vi "Generate Command Sequence.vi"() -> ()   [LabVIEW 2019]
uses:
  Controls/Command Sequene Control.ctl
panel:
  out "error out":errorcluster
  out "File path":path
  in  "Path Name":string
  out "Command Sequence":string
  in  "Auto Control":T1
  in  "Generate Path":bool
  in  "Add Command":bool
  in  "stop":bool
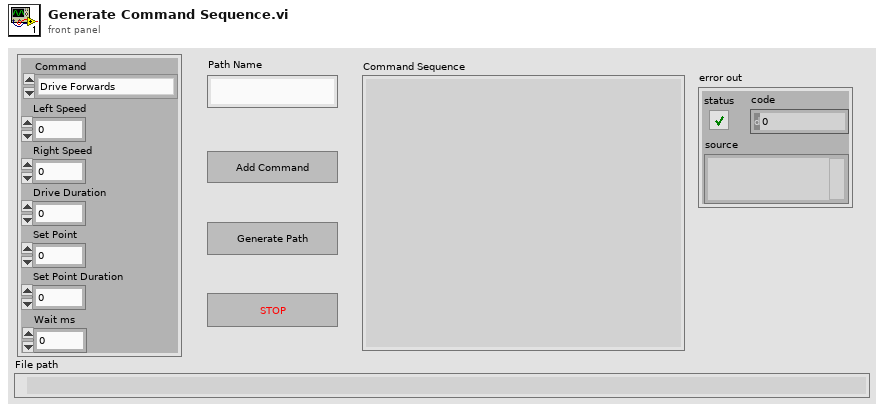
[diagram p1: front panel]
types:
  T1 = cluster{"Drive Duration":dbl, "Left Speed":dbl, "Right Speed":dbl, "Set Point":dbl, "Set Point Duration":dbl, "Command":enum16{"Drive Forwards", "Drive Backwards", "Stop", "Turn Left", "Turn Right", "Drop Intake", "Lift Intake", "Intake", "Shooter", "Transfer", "Wait"}, "Wait ms":dbl}
  T2 = typedef "Command Sequene Control.ctl" = enum16{"Idle", "Stop", "Add command", "Create Path File", "Check File Name"}
  T3 = enum16{"open", "replace", "create", "open or create", "replace or create", "replace or create with confirmation"}
  T4 = enum16{"Drive Forwards", "Drive Backwards", "Stop", "Turn Left", "Turn Right", "Drop Intake", "Lift Intake", "Intake", "Shooter", "Transfer", "Wait"}
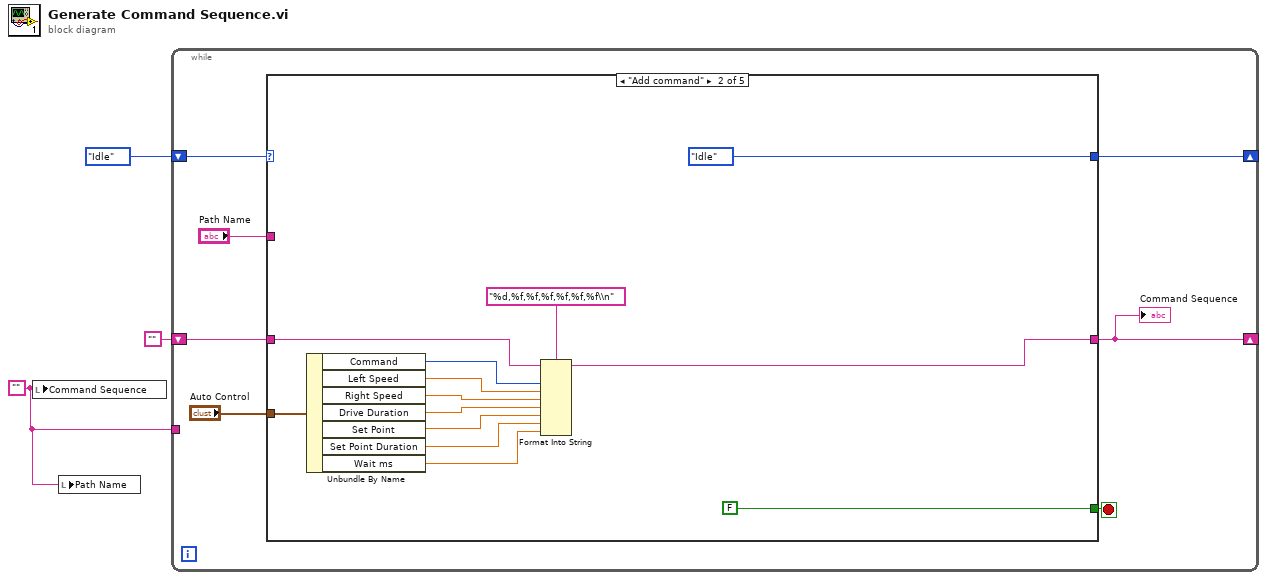
[diagram p0: block diagram]
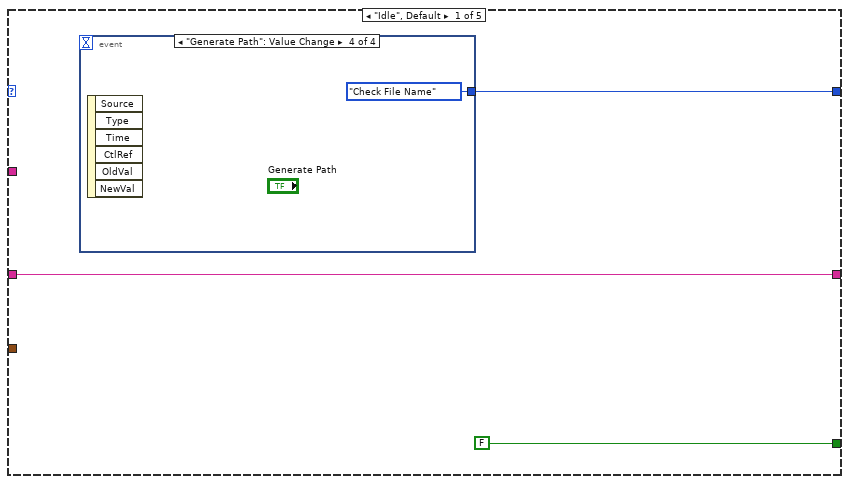
[diagram p2: hidden frame]
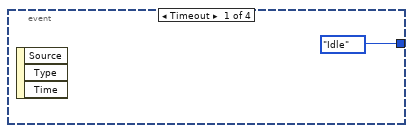
[diagram p3: hidden frame]
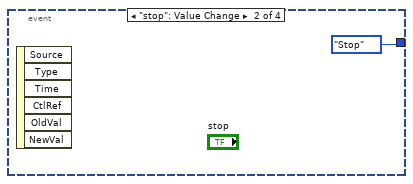
[diagram p4: hidden frame]
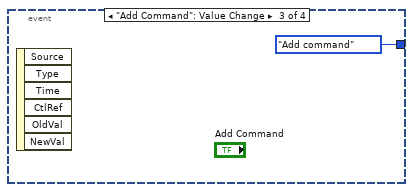
[diagram p5: hidden frame]
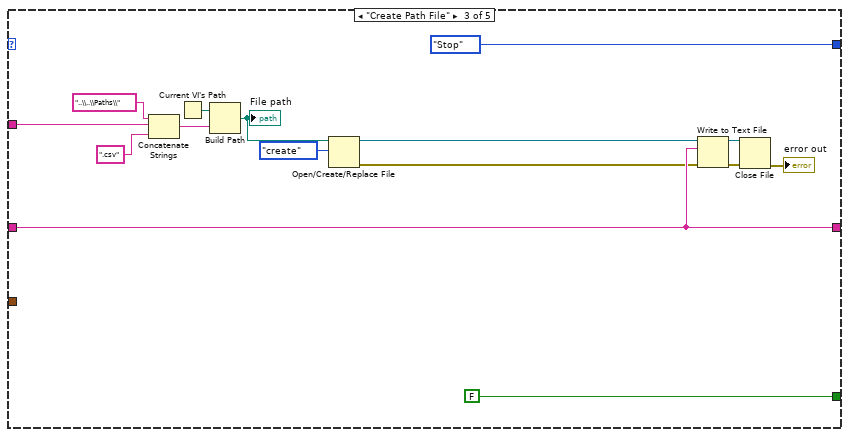
[diagram p6: hidden frame]
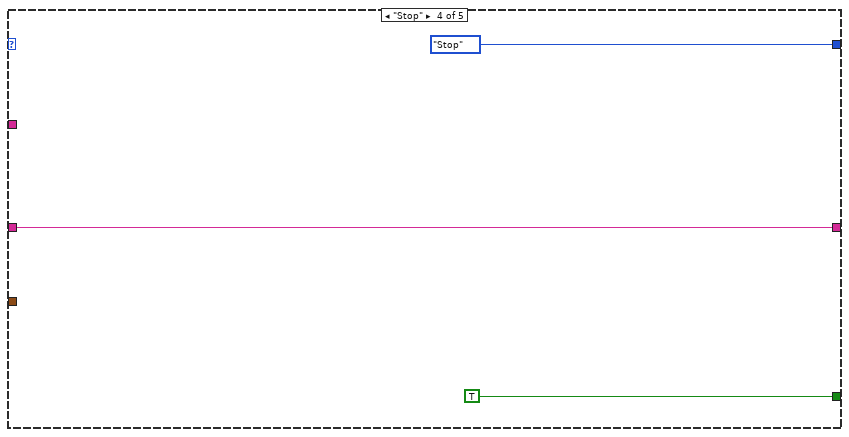
[diagram p7: hidden frame]
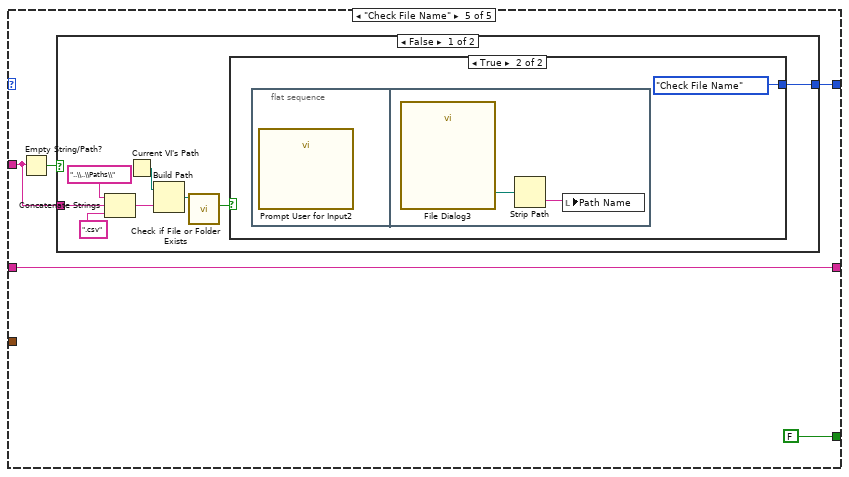
[diagram p8: hidden frame]
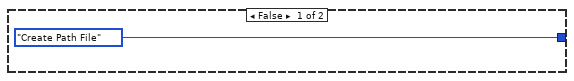
[diagram p9: hidden frame]
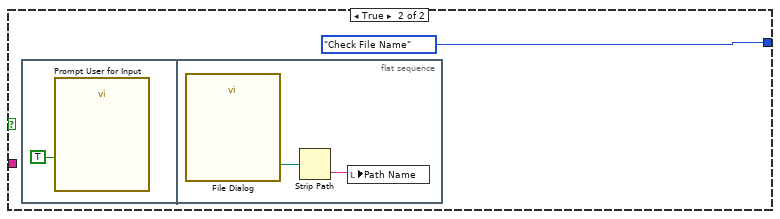
[diagram p10: hidden frame]
diagram:
  w1 = ""
  n1 = local write "Command Sequence"(w1) -> ()
  n2 = local write "Path Name"(w1) -> ()
  n3 = while {
    shift-right: [w9] -> _
    shift-left: Command_Sequene_Control."Idle" -> [w10]
    shift-right: [w5] -> _
    shift-left: "" -> [w6]
    tunnel: w1 -> [_]
    stop <- w8 stop-if-true
    n4 = case shown="\"Add command\"" w10 {
      tunnel: [w13 Command_Sequene_Control."Idle" Command_Sequene_Control."Stop" Command_Sequene_Control."Stop" w50] -> w9
      tunnel: [FALSE FALSE FALSE TRUE FALSE] -> w8
      tunnel: "Auto Control" -> [_ w28 _ _ _]
      tunnel: [w11 w19 w43 w46 w52] -> w5
      tunnel: w6 -> [w11 w20 w43 w46 w52]
      tunnel: "Path Name" -> [_ _ w31 _ w49]
      frame "Idle", Default {
        n5 = event shown="[3] \"Generate Path\": Value Change" {
          selector: _ -> [_ _ _ _]
          dyn-events: _ -> [_ _ _ _]
          timeout: _ -> [_ _ _ _]
          tunnel: [Command_Sequene_Control."Idle" Command_Sequene_Control."Stop" Command_Sequene_Control."Add command" Command_Sequene_Control."Check File Name"] -> w13
          event Timeout {
            n6 = event-data() -> ()  [unwired: 1 in, 3 out]
          }
          event "stop": Value Change {
            n7 = event-data() -> ()  [unwired: 1 in, 6 out]
          }
          event "Add Command": Value Change {
            n8 = event-data() -> ()  [unwired: 1 in, 6 out]
          }
          event "Generate Path": Value Change {
            n9 = event-data() -> ()  [unwired: 1 in, 6 out]
          }
        }
      }
      frame "Add command" {
        n10 = Unbundle By Name(w28) -> ("Command"=w26:T4, "Left Speed"=w25:dbl, "Right Speed"=w24:dbl, "Drive Duration"=w23:dbl, "Set Point"=w22:dbl, "Set Point Duration"=w21:dbl, "Wait ms"=w18:dbl)
        n11 = Format Into String(format string="%d,%f,%f,%f,%f,%f,%f\\n", initial string=w20, w26, w25, w24, w23, w22, w21, w18) -> (resulting string=w19:string)  [unwired: 1 in, 1 out]
      }
      frame "Create Path File" {
        n12 = Concatenate Strings("..\\..\\Paths\\" ("string"), w31, ".csv" ("string")) -> (w40:string)
        n13 = Current VI's Path() -> (path=w39:path)
        n14 = Build Path(base path=w39, name or relative path=w40) -> (appended path=w38:path)
        "File path" <- w38
        n15 = Open/Create/Replace File(file path (use dialog)=w38, operation (0:open)=T3."create") -> (refnum out=w34:refnum<file>, error out=w33:errorcluster)  [unwired: 4 in, 1 out]
        n16 = Write to Text File(file (use dialog)=w34, text=w43, error in=w33) -> (refnum out=w42:refnum<file>, error out=w41:errorcluster)  [unwired: 1 in, 1 out]
        n17 = Close File(refnum=w42, error in=w41) -> (error out=→"error out":errorcluster)  [unwired: 1 out]
      }
      frame "Stop" {
      }
      frame "Check File Name" {
        n18 = Empty String/Path?(string/path=w49) -> (empty?=w51:bool)
        n19 = case shown="False" w51 {
          tunnel: [w54 Command_Sequene_Control."Check File Name"] -> w50
          tunnel: w49 -> [w57 _]
          frame False {
            n20 = Concatenate Strings("..\\..\\Paths\\" ("string"), w57, ".csv" ("string")) -> (w61:string)
            n21 = Current VI's Path() -> (path=w60:path)
            n22 = Build Path(base path=w60, name or relative path=w61) -> (appended path=w56:path)
            n23 = call <vilib>:"Check if File or Folder Exists.vi"("path"=w56) -> ("file or folder exists?"=w55:bool)  [unwired: 8 in, 2 out]
            n24 = case shown="True" w55 {
              tunnel: [Command_Sequene_Control."Create Path File" Command_Sequene_Control."Check File Name"] -> w54
              frame False {
              }
              frame True {
                n25 = flat-sequence {
                  frame #0 {
                    n26 = call "Prompt User for Input2"() -> ()  [unwired: 20 in]
                  }
                  frame #1 {
                    n27 = call "File Dialog3"() -> ("selected path"=w65:path)  [unwired: 12 in, 3 out]
                    n28 = Strip Path(path=w65) -> (name=w64:string)  [unwired: 1 out]
                    n29 = local write "Path Name"(w64) -> ()
                  }
                }
              }
            }
          }
          frame True {
            n30 = flat-sequence {
              frame #0 {
                n31 = call "Prompt User for Input"("Enable"=TRUE) -> ()  [unwired: 19 in]
              }
              frame #1 {
                n32 = call "File Dialog"() -> ("selected path"=w69:path)  [unwired: 12 in, 3 out]
                n33 = Strip Path(path=w69) -> (name=w68:string)  [unwired: 1 out]
                n34 = local write "Path Name"(w68) -> ()
              }
            }
          }
        }
      }
    }
    "Command Sequence" <- w5
  }
